vi "Save_to_File_Prompt.vi"(8 "error in (no error)":errorcluster) -> (0 "error out":errorcluster, 3 "Yes":bool)   [LabVIEW 2018]
doc: "Prompts the user whether to save the file.\n\nInputs:\nError In\n\nOutputs:\nError Out;\nYes."
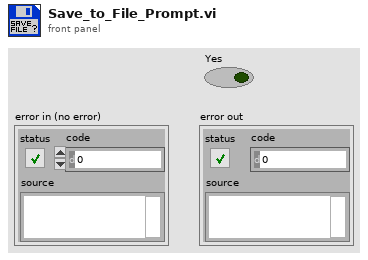
[diagram p1: front panel]
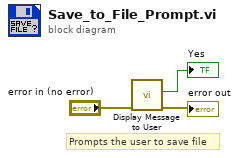
[diagram p0: block diagram]
diagram:
  # "Prompts the user to save file"
  n1 = call "Display Message to User"("error in (no error)"="error in (no error)") -> ("error out"=→"error out":errorcluster, "Yes"=→"Yes":bool)  [unwired: 9 in]
